vi "Time For Evaporation.vi"(10 "Evaporation rate":dbl, 11 "Droplet Size":dbl) -> (3 "Time for Evaporation":dbl)   [LabVIEW 2020]
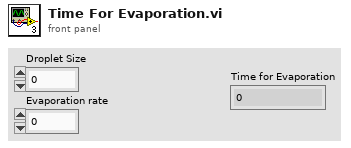
[diagram p1: front panel]
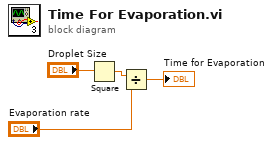
[diagram p0: block diagram]
diagram:
  n1 = Square(x="Droplet Size") -> (x^2=w4:dbl)
  n2 = Divide(x=w4, y="Evaporation rate") -> (x/y=→"Time for Evaporation":dbl)
